vi "Send Value Update.vi"(8 "error in (no error)":errorcluster, 9 "Value":variant, 10 "Datum Name":string, 11 "IViewable in":refnum<class "IViewable.lvclass">) -> (0 "error out":errorcluster)   [LabVIEW 2017, in "IViewable.lvlib" / "IViewable.lvclass"]
uses:
  IViewable.lvclass
  C:/Program Files (x86)/National Instruments/LabVIEW 2017/vi.lib/ActorFramework/Actor/Actor.lvclass
  <vilib>/ActorFramework/Actor/Actor.lvclass/Actor.ctl
  IViewable Messages/Catch Nested Value Change Msg/Nested Value Update Msg.lvclass/Nested Value Update Msg.ctl
  <vilib>/ActorFramework/Message Enqueuer/Message Enqueuer.lvclass/Message Enqueuer.ctl
  <vilib>/ActorFramework/Message Enqueuer/Enqueue.vi
  IViewable Messages/Catch Nested Value Change Msg/Nested Value Update Msg.lvclass
  C:/Program Files (x86)/National Instruments/LabVIEW 2017/vi.lib/ActorFramework/Message/Message.lvclass
  <vilib>/ActorFramework/Message Priority Queue/Priority Enqueue.vi
  <vilib>/ActorFramework/Actor/Actor.lvclass
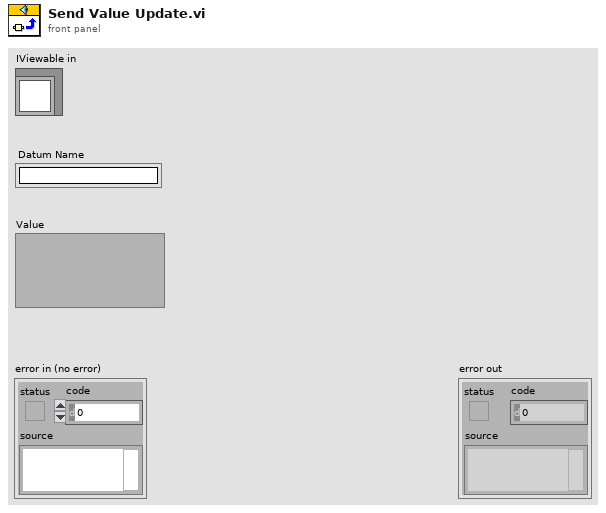
[diagram p1: front panel]
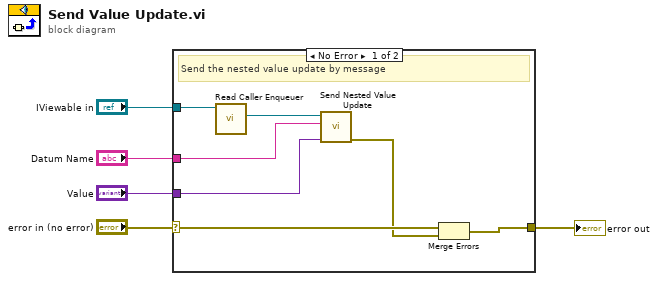
[diagram p0: block diagram]
diagram:
  n1 = case shown="No Error" "error in (no error)" {
    selector: "error in (no error)" -> [w10 w13]
    tunnel: "IViewable in" -> [w12 _]
    tunnel: [w9 w13] -> w3
    tunnel: "Datum Name" -> [w7 _]
    tunnel: "Value" -> [w6 _]
    frame No Error {
      # "Send the nested value update by message"
      n2 = call <vilib>:"Read Caller Enqueuer.vi"("Actor"=w12) -> ("Caller Enqueuer"=w11:refnum<class "Message Enqueuer.lvclass">)  [unwired: 10 in]
      n3 = call "Send Nested Value Update.vi"("Value"=w6, "Datum Name"=w7, "Message Enqueuer"=w11) -> ("error out"=w8:errorcluster)  [unwired: 7 in, 1 out]
      n4 = Merge Errors(w10, w8) -> (w9:errorcluster)
    }
    frame Error {
      # "Do not send on error"
    }
  }
  "error out" <- w3
